vi "LED Buffer Manager.vi"(7 "action":T1(ring), 8 "Colors":u32[](array[colorbox]), 9 "length":i32, 10 "startIndex":i32, 11 "deviceIndex":i32) -> ()   [LabVIEW 2026]
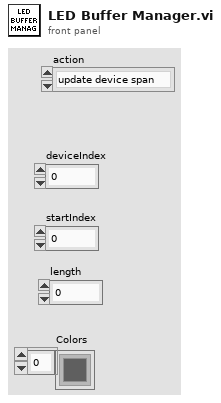
[diagram p1: front panel]
types:
  T1 = enum16{"update device span", "update LED buffer", "clear"}
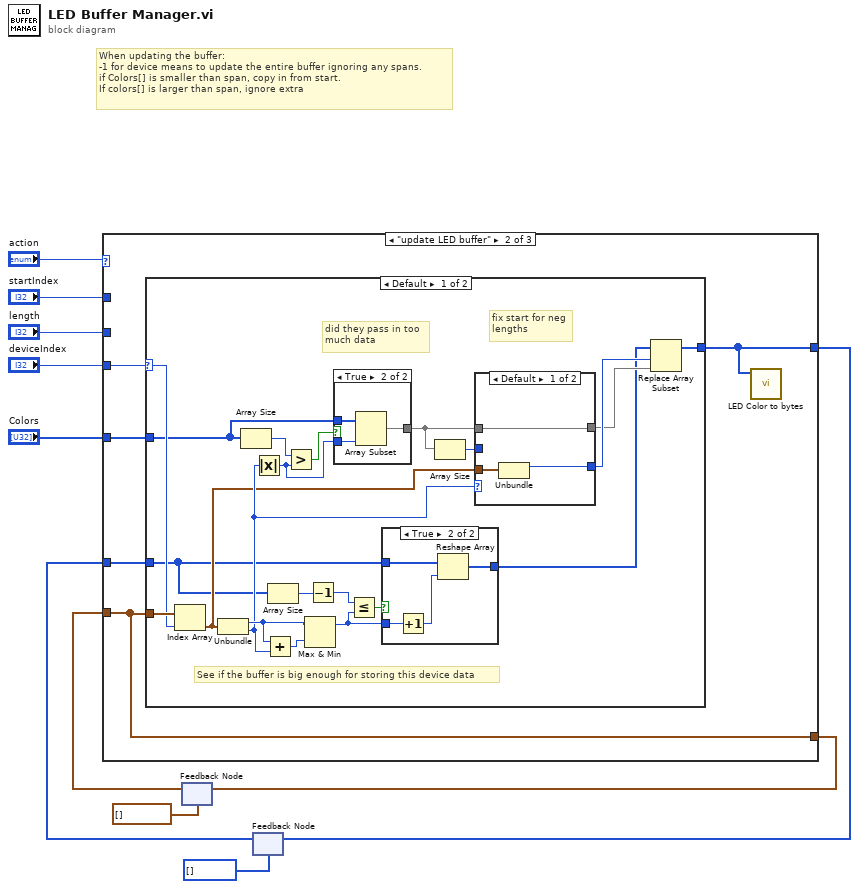
[diagram p0: block diagram]
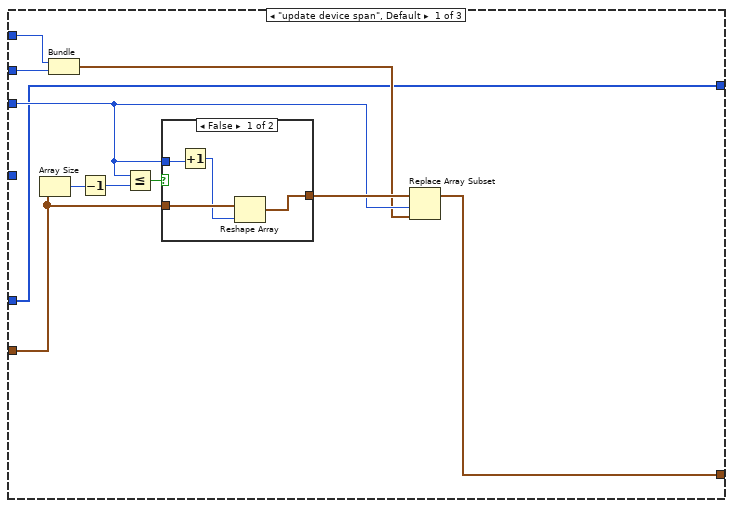
[diagram p2: hidden frame]
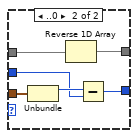
[diagram p4: hidden frame]
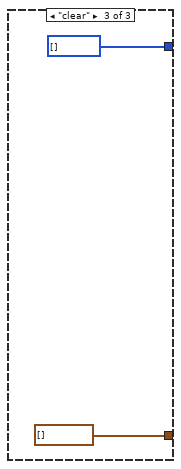
[diagram p8: hidden frame]
diagram:
  # "When updating the buffer:\n-1 for device means to update the entire buffer ignoring any spans.\nif Colors[] is smaller than span, copy in from start.\nIf colors[] is larger than span, ignore extra"
  n1 = feedback #1(cluster{"index":i32, "length":i32}[] []) -> (w10:cluster{"index":i32, "length":i32}[])
  n2 = feedback #2(u32[] [] ("Colors")) -> (w2:u32[])
  n3 = case shown="\"update LED buffer\"" "action" {
    tunnel: w10 -> [w17 w29 _]
    tunnel: [w13 w29 cluster{"index":i32, "length":i32}[] []] -> w9
    tunnel: "length" -> [w22 _ _]
    tunnel: "startIndex" -> [w21 _ _]
    tunnel: "deviceIndex" -> [w15 w32 _]
    tunnel: "Colors" -> [_ w31 _]
    tunnel: [w12 w28 u32[] [] ("Colors")] -> w3
    tunnel: w2 -> [w12 w30 _]
    frame "update device span", Default {
      n4 = Array Size(array=w17) -> (size(s)=w20:i32)
      n5 = Bundle("startIndex"=w21, "length"=w22) -> (w14:cluster{"startIndex":i32, "length":i32})  [unwired: 1 in]
      n6 = Decrement(x=w20) -> (x-1=w19:i32)
      n7 = Less Or Equal?(x=w15, y=w19) -> (x <= y?=w18:bool)
      n8 = case shown="False" w18 {
        tunnel: w17 -> [w26 w27]
        tunnel: w15 -> [w25 _]
        tunnel: [w23 w27] -> w16
        frame False {
          n9 = Increment(x=w25) -> (x+1=w24:i32)
          n10 = Reshape Array(w26, w24) -> (w23:cluster{"index":i32, "length":i32}[])
        }
        frame True {
        }
      }
      n11 = Replace Array Subset(array=w16, new element=w14, index=w15) -> (w13:cluster{"index":i32, "length":i32}[])
    }
    frame "update LED buffer" {
      n12 = case shown="Default" w32 {
        selector: w32 -> [w52 _]
        tunnel: [w51 w72] -> w28
        tunnel: w31 -> [w43 w72]
        tunnel: w30 -> [w34 _]
        tunnel: w29 -> [w53 _]
        frame Default {
          # "did they pass in too\nmuch data"
          # "fix start for neg\nlengths"
          # "See if the buffer is big enough for storing this device data"
          n13 = Index Array(array=w53, index=w52) -> (element=w39:cluster{"index":i32, "length":i32})
          n14 = Unbundle(w39) -> ("index"=w49:i32, "length"=w40:i32)
          n15 = Array Size(array=w43) -> (size(s)=w44:i32)
          n16 = Absolute Value(x=w40) -> (abs(x)=w42:i32)
          n17 = Add(x=w49, y=w40) -> (x+y=w50:i32)
          n18 = Array Size(array=w34) -> (size(s)=w48:i32)
          n19 = Greater?(x=w44, y=w42) -> (0:w41:bool)
          n20 = Max & Min(x=w49, y=w50) -> (max(x,y)=w46:i32)  [unwired: 1 out]
          n21 = Decrement(x=w48) -> (x-1=w47:i32)
          n22 = case shown="True" w41 {
            tunnel: w43 -> [w63 w66]
            tunnel: w42 -> [_ w65]
            tunnel: [w63 w64] -> w38
            frame False {
            }
            frame True {
              n23 = Array Subset(array=w66, length=w65) -> (w64:u32[])  [unwired: 1 in]
            }
          }
          n24 = Less Or Equal?(x=w47, y=w46) -> (x <= y?=w45:bool)
          n25 = case shown="True" w45 {
            tunnel: w34 -> [w67 w71]
            tunnel: w46 -> [_ w70]
            tunnel: [w67 w68] -> w33
            frame False {
            }
            frame True {
              n26 = Increment(x=w70) -> (x+1=w69:i32)
              n27 = Reshape Array(w71, w69) -> (w68:u32[])
            }
          }
          n28 = Array Size(array=w38) -> (size(s)=w37:i32)
          n29 = case shown="Default" w40 {
            tunnel: w38 -> [w56 w62]
            tunnel: [w56 w61] -> w35
            tunnel: w39 -> [w55 w60]
            tunnel: w37 -> [_ w57]
            tunnel: [w54 w58] -> w36
            frame Default {
              n30 = Unbundle(w55) -> ("index"=w54:i32)  [unwired: 1 out]
            }
            frame ..0 {
              n31 = Unbundle(w60) -> ("index"=w59:i32)  [unwired: 1 out]
              n32 = Reverse 1D Array(array=w62) -> (reversed array=w61:u32[])
              n33 = Subtract(x=w59, y=w57) -> (x-y=w58:i32)
            }
          }
          n34 = Replace Array Subset(array=w33, new element=w35, index=w36) -> (w51:u32[])
        }
        frame -1 {
        }
      }
      n35 = call "LED Color to bytes.vi"("Array"=w28) -> ()  [unwired: 11 in]
    }
    frame "clear" {
    }
  }
  n36 = feedback-in #1(w9) -> ()
  n37 = feedback-in #2(w3) -> ()
